vi "PID_screen_V2.0.vi"() -> ()   [LabVIEW 2022 SP3]
panel:
  out "Countdown Timer (CDT)":dbl format="T%<+%H:%M:%S%3u>t"
  out "Date":timestamp format="%<%d/%m/%Y>T"
  in  "Close":bool
  in  "Screen No":dbl
  out "Indian Standard Time (IST)":timestamp format="%<%H:%M:%S%2u>T"
  out "B_LO_PV_05_HSS":bool
  out "B_LO_PV_05":bool caption="Boolean"
  out "B_GN_PV_02_HSS":bool
  out "B_GN_PV_02":bool caption="Boolean"
  out "B_GN_PV_07_HSS":bool
  out "B_GN_PV_07":bool caption="Boolean"
  out "LOX_31KL_Tank":dbl(slide) scale=0.0..300.0
  out "B_GN_PV_03_HSS":bool
  out "B_GN_PV_03":bool caption="Boolean"
  out "B_GN_PV_04_HSS":bool
  out "B_GN_PV_04":bool caption="Boolean"
  out "B_GN_P_32":dbl format="%.2f bar"
  out "B_GN_PV_09_HSS":bool
  out "B_GN_PV_09":bool caption="Boolean"
  out "B_GN_P_05":dbl format="%.2f bar"
  out "B_GN_PV_08_HSS":bool
  out "B_GN_PV_08":bool caption="Boolean"
  out "B_GN_P_04":dbl format="%.2f bar"
  out "B_GN_P_03":dbl format="%.2f bar"
  out "B_GN_CV_01":dbl format="%.0f %%"
  out "B_GN_CV_01":bool caption="Boolean"
  out "B_GN_P_09":dbl format="%.2f bar"
  out "B_GN_P_10":dbl format="%.2f bar"
  out "B_GN_P_08":dbl format="%.2f bar"
  out "B_GN_P_07":dbl format="%.2f bar"
  out "B_GO_P_04":dbl format="%.2f bar"
  out "B_GN_P_06":dbl format="%.2f bar"
  out "B_GN_P_01":dbl format="%.2f bar"
  out "B_GN_P_02":dbl format="%.2f bar"
  out "B_GN_P_33":dbl format="%.2f bar"
  out "B_GO_P_02":dbl format="%.2f bar"
  out "B_GO_P_03":dbl format="%.2f bar"
  out "B_GO_P_01":dbl format="%.2f bar"
  out "B_GN_P_13":dbl format="%.2f bar"
  out "B_GN_T_01":dbl format="%.2f bar"
  out "B_GN_P_12":dbl format="%.2f bar"
  out "B_GN_P_11":dbl format="%.2f bar"
  out "B_LO_PV_09_HSS":bool
  out "B_LO_PV_09":bool caption="Boolean"
  out "B_LO_PV_HSS":bool
  out "B_LO_PV":bool caption="Boolean"
  out "B_LO_P_10":dbl format="%.2f bar"
  out "B_LO_PV_01_HSS":bool
  out "B_LO_PV_01":bool caption="Boolean"
  out "B_GN_PV_07_HSS 2":bool
  out "B_GN_PV_07 2":bool caption="Boolean"
  out "B_LO_PV_02_HSS":bool
  out "B_LO_PV_02":bool caption="Boolean"
  out "B_LO_FM_03":dbl format="%.2f Kg/s"
  out "B_LO_T_03":dbl format="%.2f bar"
  out "B_LO_P_03":dbl format="%.2f bar"
  out "B_LO_P_09":dbl format="%.2f bar"
  out "B_LO_PV_04_HSS":bool
  out "B_LO_PV_04":bool caption="Boolean"
  out "B_LO_FM_02":dbl format="%.2f Kg/s"
  out "B_LO_P_06":dbl format="%.2f bar"
  out "B_HE_T_03":dbl format="%.2f bar"
  out "B_LO_T_06":dbl format="%.2f bar"
  out "B_LO_PV_13_HSS":bool
  out "B_LO_PV_13":bool caption="Boolean"
  out "B_LO_PV_06_HSS":bool
  out "B_LO_PV_06":bool caption="Boolean"
  out "B_LO_PV_08_HSS":bool
  out "B_LO_PV_08":bool caption="Boolean"
  out "B_LO_PV_07_HSS":bool
  out "B_LO_PV_07":bool caption="Boolean"
  out "B_LO_PV_10_HSS":bool
  out "B_LO_PV_10":bool caption="Boolean"
  out "B_LO_PV_11_HSS":bool
  out "B_LO_PV_11":bool caption="Boolean"
  out "B_LO_PV_12_HSS":bool
  out "B_LO_PV_12":bool caption="Boolean"
  out "B_LO_PV_03_HSS":bool
  out "B_LO_PV_03":bool caption="Boolean"
  out "B_LO_FM_01":dbl format="%.2f Kg/s"
  out "B_LO_P_08":dbl format="%.2f bar"
  out "B_LO_T_01":dbl format="%.2f bar"
  out "B_LO_P_01":dbl format="%.2f bar"
  out "B_HE_P_04":dbl format="%.2f bar"
  out "B_HE_P_03":dbl format="%.2f bar"
  out "B_HE_T_02":dbl format="%.2f bar"
  out "B_HE_P_02":dbl format="%.2f bar"
  out "B_HE_P_01":dbl format="%.2f bar"
  out "B_HE_T_01":dbl format="%.2f bar"
  out "B_GN_PV_07_HSS":bool
  out "B_GN_PV_07":bool caption="Boolean"
  out "B_LN_T_03":dbl format="%.2f bar"
  out "B_LN_P_08":dbl format="%.2f bar"
  out "B_LO_T_04":dbl format="%.2f bar"
  out "B_LO_P_04":dbl format="%.2f bar"
  out "B_LO_T_05":dbl format="%.2f bar"
  out "B_LO_P_05":dbl format="%.2f bar"
  out "B_LO_T_02":dbl format="%.2f bar"
  out "B_LO_P_02":dbl format="%.2f bar"
  out "B_LO_P_07":dbl format="%.2f bar"
  out "B_LO_P_11":dbl format="%.2f bar"
  # "BSTF PID SCREEN"
  # "VERSION 2.0"
  # "Connect to all stage\nLOX and LIN EV"
  # "Stage Cryo Valves Command"
  # "Connect to all ground\nLOX and LIN EV"
  # "LOX/LIN Ground Valves Command"
  # "GOX Ignitor Purge"
  # "To Atmosphere"
  # "Engine LOX Injector Purge"
  # "LOX/LIN Feed Line Purge"
  # "LOX Tank Pressurization"
  # "Connected to\nStage COPV \nUbmilical"
  # "LOX Tank\nVent"
  # "LOX\n31KL\nTANK"
  # "LOX PUMP SEAL PURGE"
  # "ENGINE"
  # "GOX IGNITOR PURGE"
  # "GOX MANIFOLD"
  # "LOX\nFILL"
  # "GN2\nVaporiser\nSource"
  # "B_LO_SP_01"
  # "BOOSTER PUMP"
  # "GOX\nSource"
  # "Common\nGN2\nSource"
  # "GHe\nSource"
  # "LOX CLUSTER MANIFOLD"
  # "TO STAGE FILL/DRAIN"
  # "STAGE SUBCOOL RETURN"
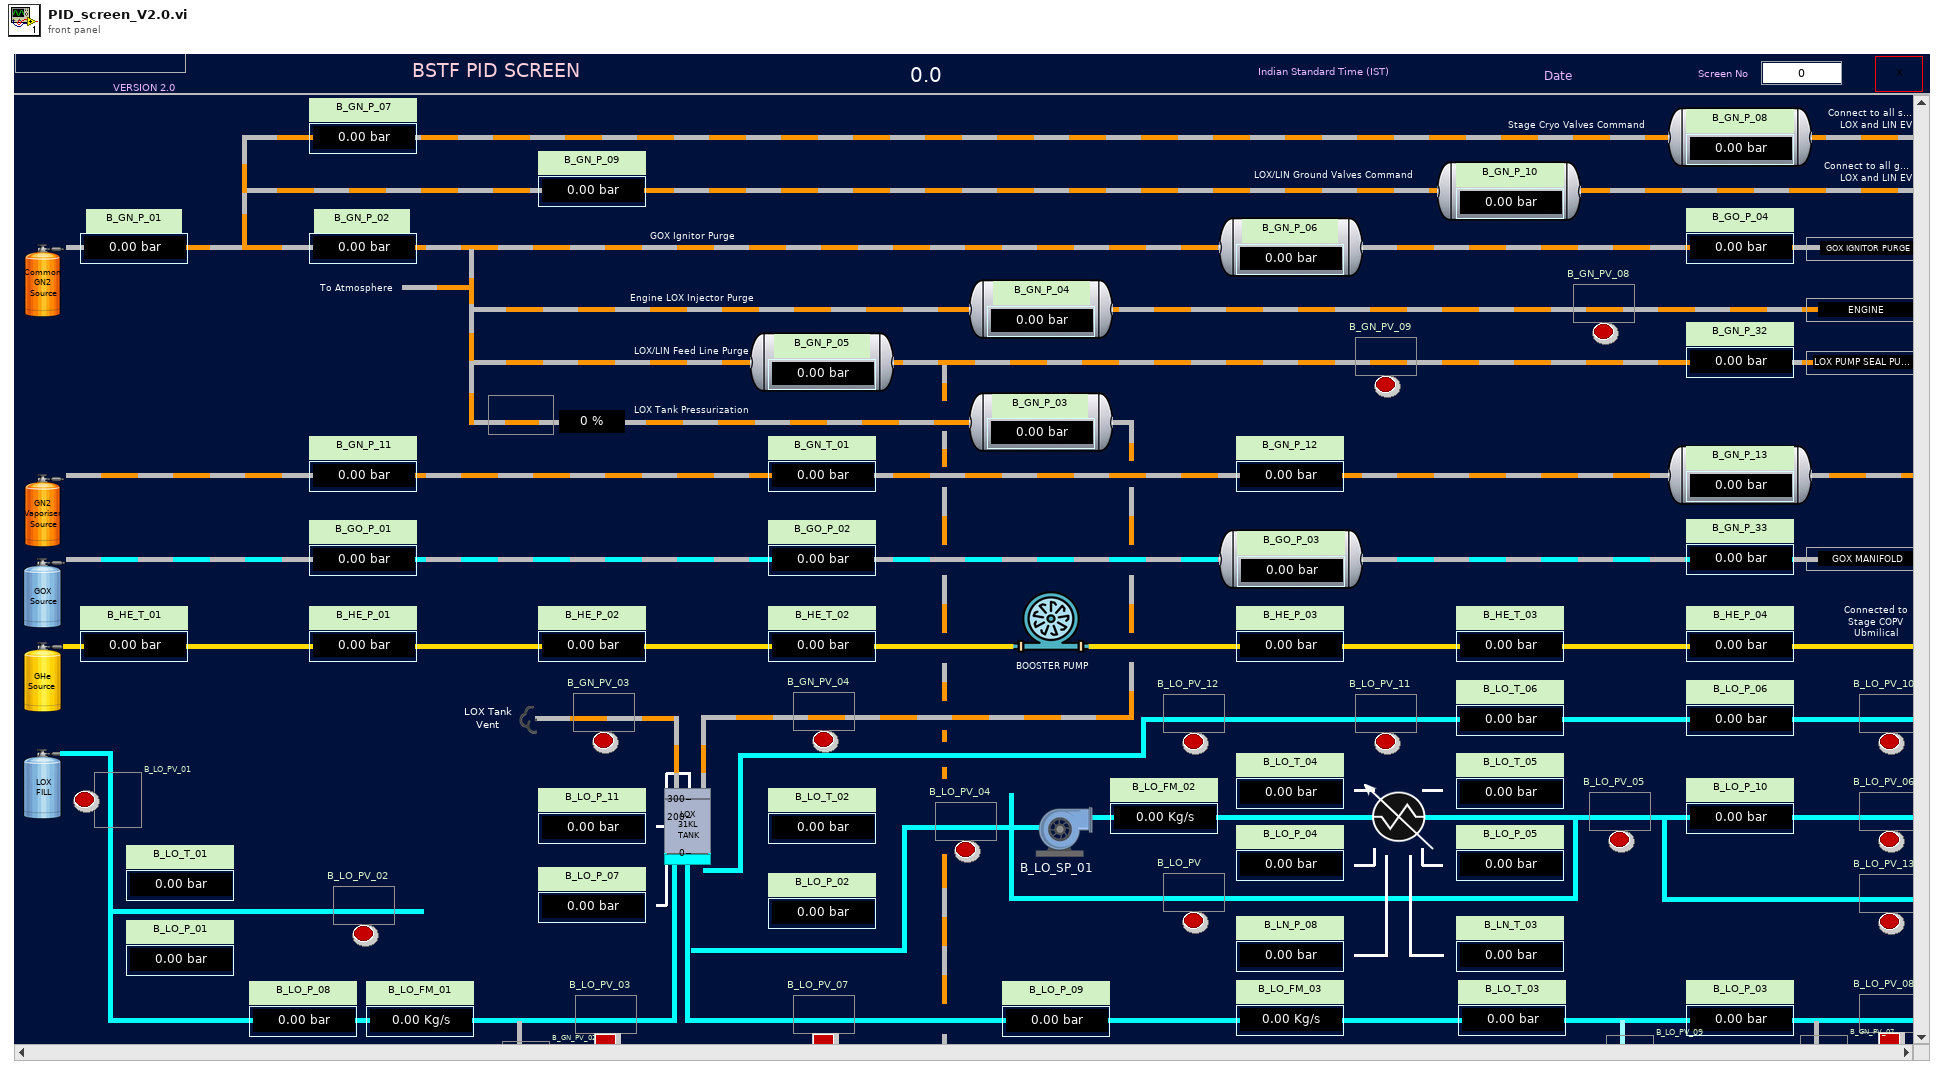
[diagram p1: front panel]
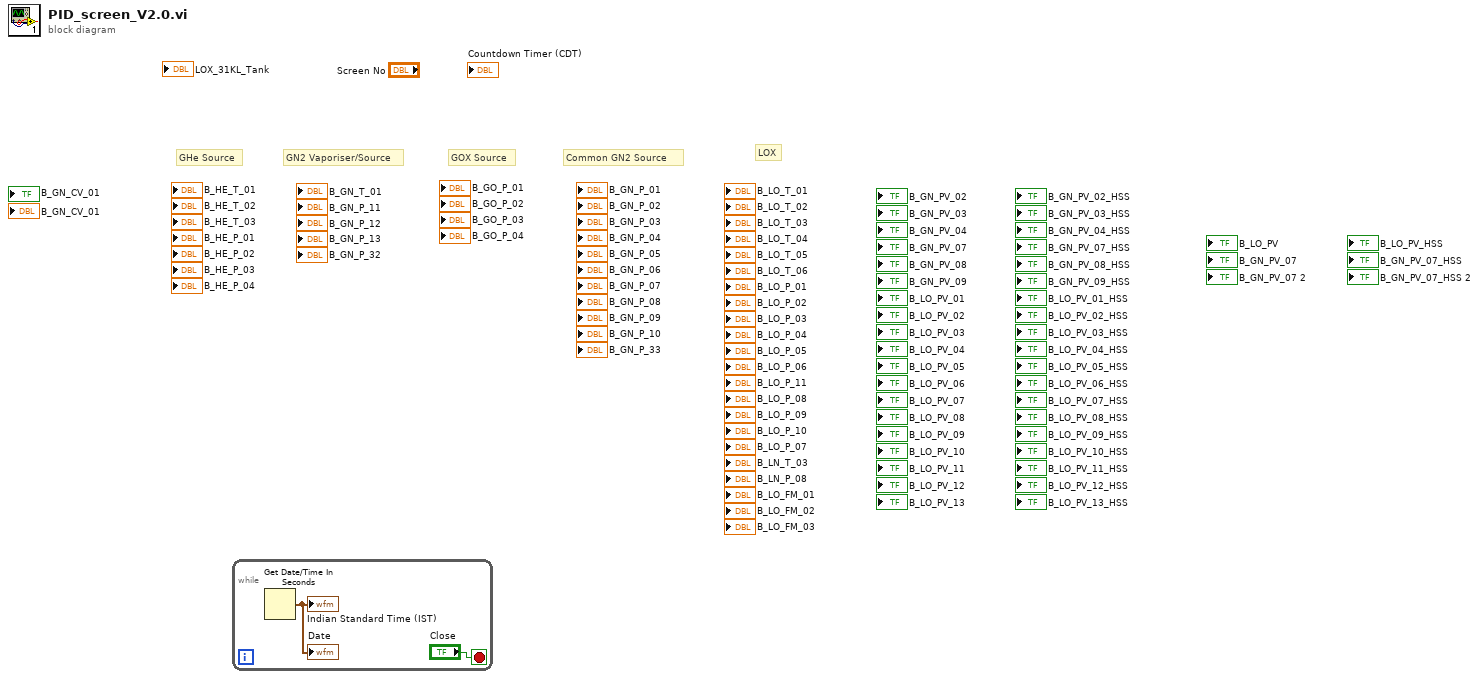
[diagram p0: block diagram]
diagram:
  # "LOX"
  # "Common GN2 Source"
  # "GOX Source"
  # "GN2 Vaporiser/Source"
  # "GHe Source"
  n1 = while {
    stop <- "Close" stop-if-true
    n2 = Get Date/Time In Seconds() -> (seconds since 1Jan1904=→"Indian Standard Time (IST)" →"Date":timestamp)
  }
